vi "serial_write_and_wait.vi"(2 "error in (no error)":errorcluster, 3 "write buffer":string, 4 "serial in":refnum<visa-resource-name>) -> (0 "error out":errorcluster, 1 "serial out":refnum<visa-resource-name>)   [LabVIEW 2016]
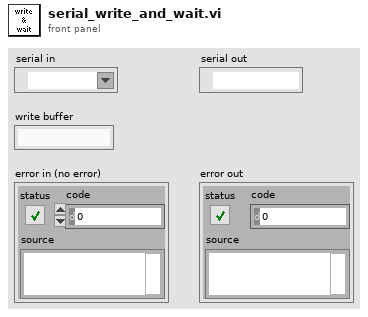
[diagram p1: front panel]
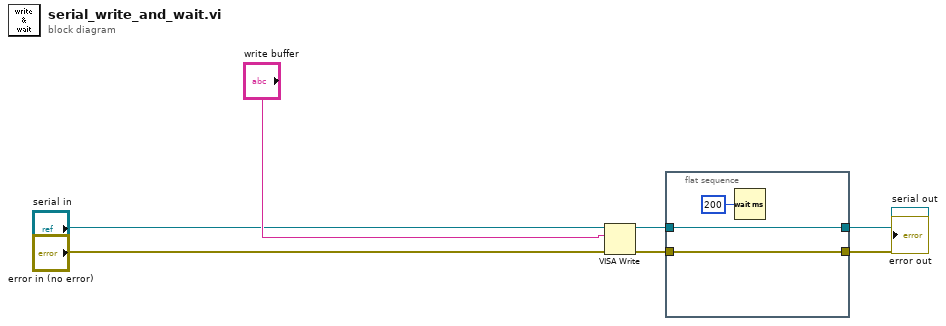
[diagram p0: block diagram]
diagram:
  n1 = VISA Write(VISA resource name="serial in", write buffer="write buffer", error in (no error)="error in (no error)") -> (VISA resource name out=w5:refnum<visa-resource-name>, error out=w4:errorcluster)  [unwired: 1 out]
  n2 = flat-sequence {
    tunnel: [w10] -> w7
    tunnel: w4 -> [w10]
    tunnel: [w9] -> w6
    tunnel: w5 -> [w9]
    frame #0 {
      n3 = Wait (ms)(milliseconds to wait=u32 200) -> ()  [unwired: 1 out]
    }
  }
  "error out" <- w7
  "serial out" <- w6
